vi "CC Observation Insert Airmass in Table.vi"(9 "Airmass Idx":i32, 10 "Air Mass":T1[](array[typedef]), 11 "Table":string[][](array[string])) -> (3 "Table out":string[][](array[string]))   [LabVIEW 2024]
uses:
  CC cluster Air Mass Data.ctl
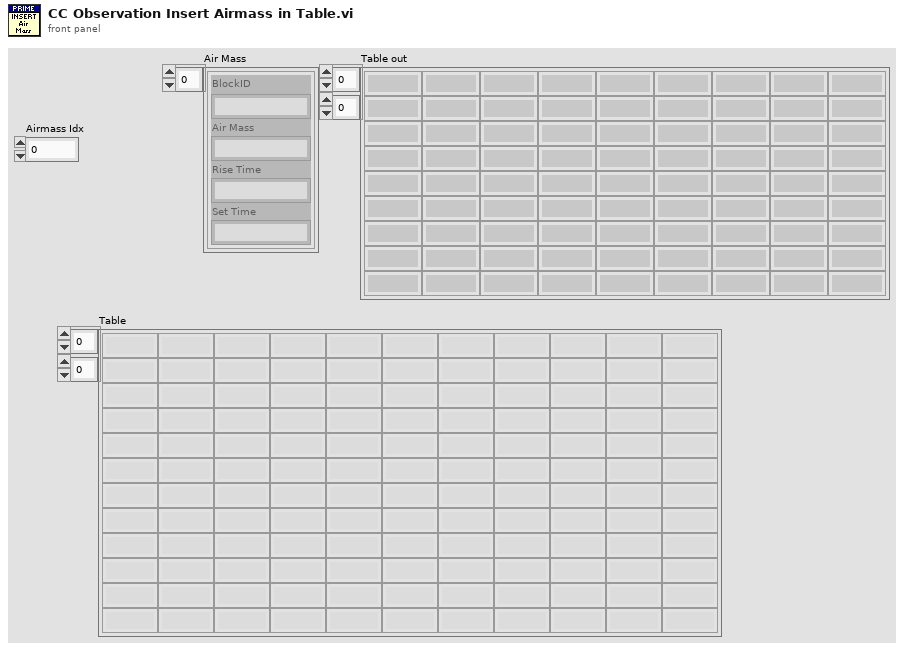
[diagram p1: front panel]
types:
  T1 = typedef "CC cluster Air Mass Data.ctl" = cluster{"BlockID":string, "Air Mass":string, "Rise Time":string, "Set Time":string}
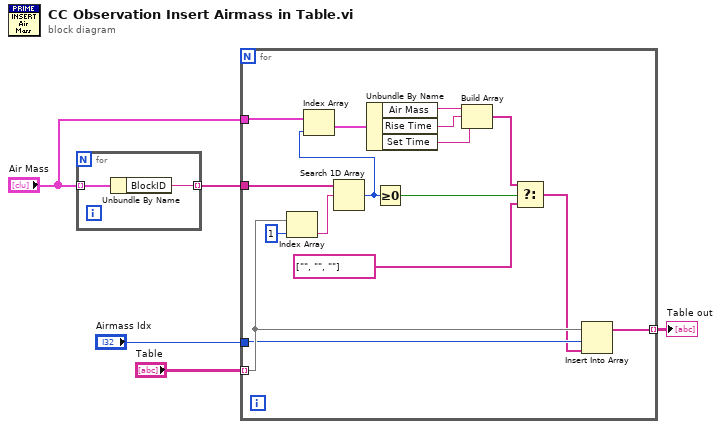
[diagram p0: block diagram]
diagram:
  n1 = for {
    tunnel: "Air Mass" -> [w7] mode=indexing
    tunnel: [w6] -> w3 mode=indexing
    n2 = Unbundle By Name(w7) -> ("BlockID"=w6:string)
  }
  n3 = for {
    tunnel: "Airmass Idx" -> [w16]
    tunnel: "Table" -> [w17] mode=indexing
    tunnel: w3 -> [w20]
    tunnel: "Air Mass" -> [w18]
    tunnel: [w11] -> w1 mode=indexing
    n4 = Index Array(array=w17, index=1) -> (element=w19:string)
    n5 = Search 1D Array(1D array=w20, element=w19) -> (index of element=w8:i32)  [unwired: 1 in]
    n6 = Index Array(array=w18, index=w8) -> (element=w9:T1)
    n7 = Unbundle By Name(w9) -> ("Air Mass"=w23:string, "Rise Time"=w22:string, "Set Time"=w21:string)
    n8 = Greater Or Equal To 0?(x=w8) -> (x >= 0?=w15:bool)
    n9 = Build Array(w23, w22, w21) -> (w14:string[])
    n10 = Select(t=w14, s=w15, f=string[] ["", "", ""]) -> (s? t:f=w12:string[])
    n11 = Insert Into Array(array=w17, index=w16, new element=w12) -> (w11:string[])
  }
  "Table out" <- w1
